vi "conveyor valve.vi"() -> ()   [LabVIEW 2016]
panel:
  in  "?":bool
  in  "Reset":bool
  in  "Selector":bool
  out "?":bool
  out "?":bool
  out "?":bool
  out "started":bool
  out "conveyor":dbl(slide) scale=0.0..100.0
  # "Start"
  # "Stop"
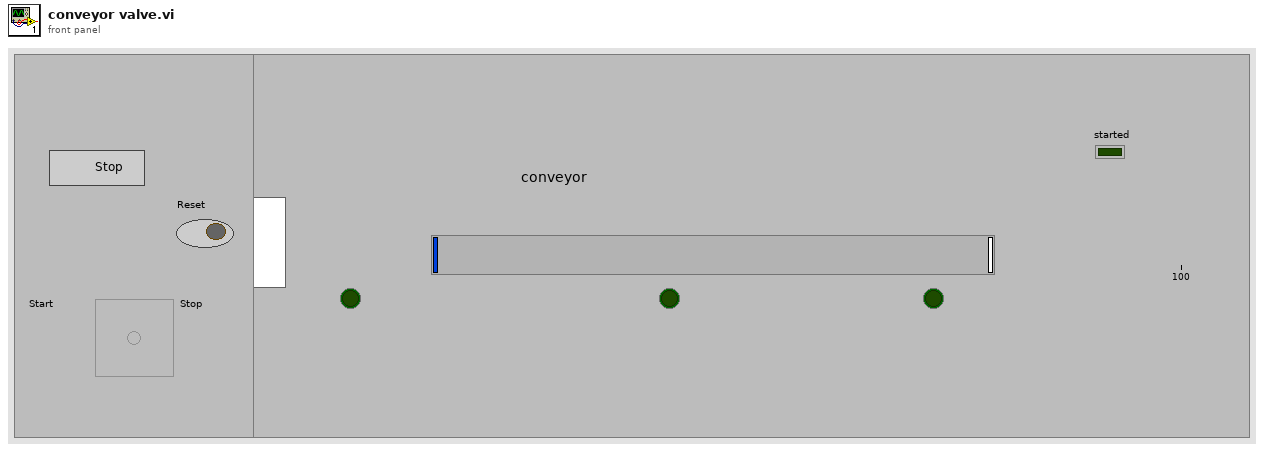
[diagram p1: front panel]
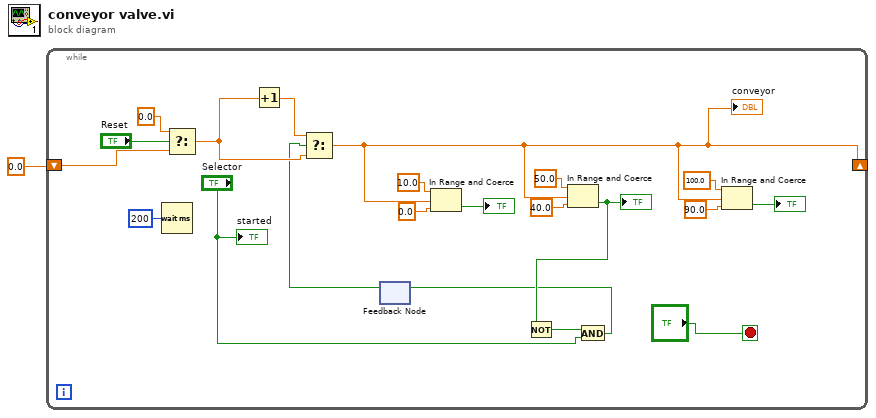
[diagram p0: block diagram]
diagram:
  n1 = while {
    shift-right: [w8] -> _
    shift-left: 0.0 -> [w20]
    stop <- "?" stop-if-true
    n2 = Wait (ms)(milliseconds to wait=u32 200) -> ()  [unwired: 1 out]
    n3 = Select(t=0.0, s="Reset", f=w20) -> (s? t:f=w17:dbl)
    n4 = Increment(x=w17) -> (x+1=w18:dbl)
    n5 = feedback #1() -> (w2:bool)  [unwired: 1 in]
    n6 = Select(t=w18, s=w2, f=w17) -> (s? t:f=w8:dbl)
    "conveyor" <- w8
    n7 = In Range and Coerce(upper limit=10.0, x=w8, lower limit=0.0) -> (In Range?=→"?":bool)  [unwired: 1 out]
    n8 = In Range and Coerce(upper limit=50.0, x=w8, lower limit=40.0) -> (In Range?=w4:bool)  [unwired: 1 out]
    "?" <- w4
    n9 = Not(x=w4) -> (.not. x?=w6:bool)
    n10 = And(x=w6, y="Selector") -> (x .and. y?=w3:bool)
    n11 = feedback-in #1(w3) -> ()
    n12 = In Range and Coerce(upper limit=100.0, x=w8, lower limit=90.0) -> (In Range?=→"?":bool)  [unwired: 1 out]
    "started" <- "Selector"
  }
